vi "Append Waveform Properties to TDMS Channels.vi"(8 "error in":errorcluster, 10 "File Log Spec In":T1 {"File Node Ref" format="%.0x"}, 11 "TDMS File In":refnum<k34>) -> (0 "error out":errorcluster, 2 "File Log Spec":T1 {"File Node Ref" format="%.0x"}, 3 "TDMS File Out":refnum<k34>)   [LabVIEW 2027, in "Embedded Data Logger Engine.lvlib"]
uses:
  Embedded Data Logger Engine.lvlib
  File Logging Specification.ctl
  Group Logging Specification.ctl
  Group Buffer Data.ctl
  Property Specification.ctl
  <vilib>/NI VeriStand/Custom Device API/Custom Device Item Ref.ctl
  Shared/Segment Files By.ctl
  Logging State.ctl
  <vilib>/NI VeriStand/Custom Device API/Custom Device API.lvlib
  Shared/Embedded Data Logger Shared.lvlib
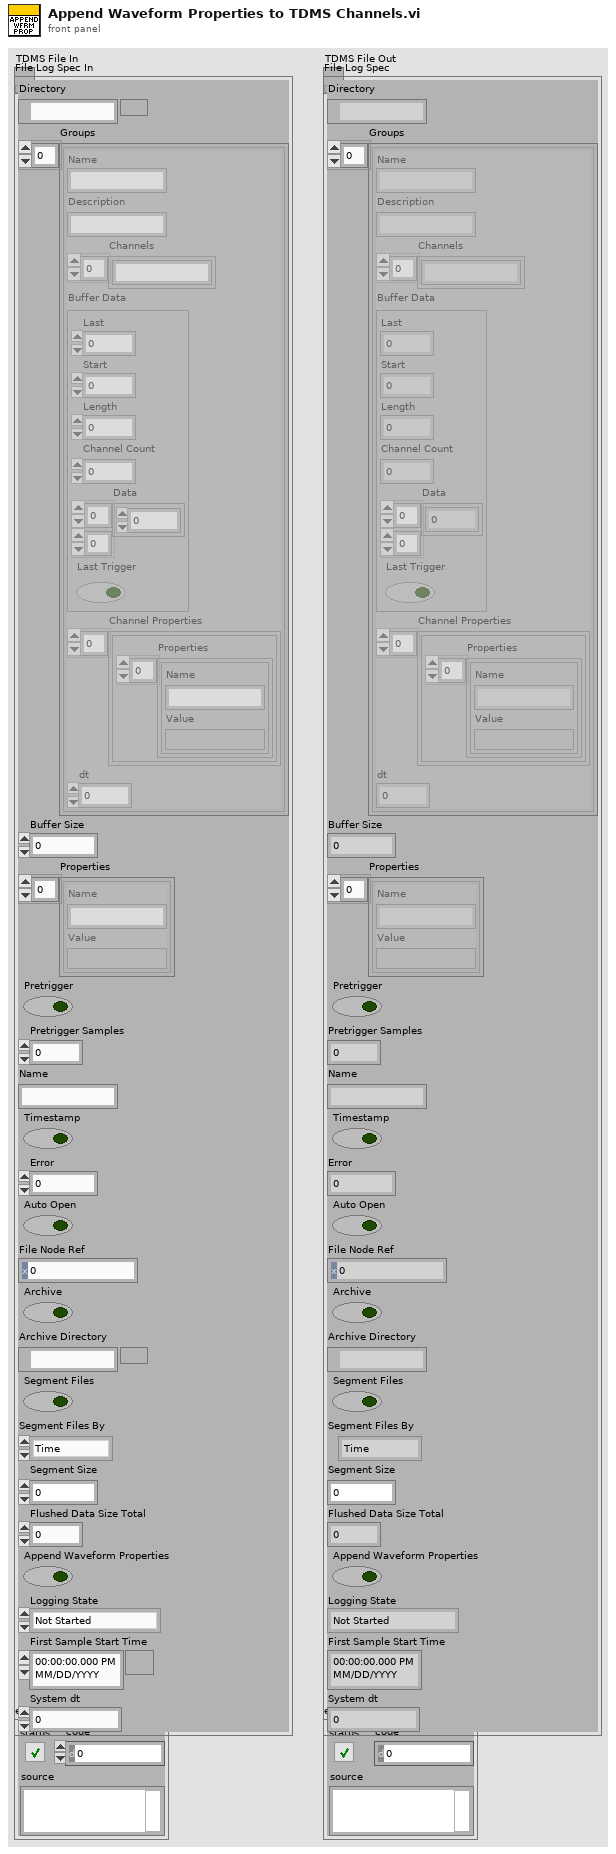
[diagram p1: front panel]
types:
  T1 = typedef "Embedded Data Logger Engine.lvlib/File Logging Specification.ctl" = cluster{"Directory":path, "Groups":T2[], "Buffer Size":i32, "Properties":T4[], "Pretrigger":bool, "Pretrigger Samples":i32, "Name":string, "Timestamp":bool, "Error":i32, "Auto Open":bool, "File Node Ref":T5, "Archive":bool, "Archive Directory":path, "Segment Files":bool, "Segment Files By":T6, "Segment Size":u32, "Flushed Data Size Total":u32, "Append Waveform Properties":bool, "Logging State":T7, "First Sample Start Time":timestamp, "System dt":dbl}
  T2 = typedef "Embedded Data Logger Engine.lvlib/Group Logging Specification.ctl" = cluster{"Name":string, "Description":string, "Channels":string[], "Buffer Data":T3, "Channel Properties":cluster{"Properties":T4[]}[], "dt":dbl}
  T3 = typedef "Embedded Data Logger Engine.lvlib/Group Buffer Data.ctl" = cluster{"Last":i32, "Start":i32, "Length":i32, "Channel Count":i32, "Data":dbl[][], "Last Trigger":bool}
  T4 = typedef "Embedded Data Logger Engine.lvlib/Property Specification.ctl" = cluster{"Name":string, "Value":variant}
  T5 = typedef "Custom Device API.lvlib/Custom Device Item Ref.ctl" = u64
  T6 = typedef "Embedded Data Logger Shared.lvlib/Segment Files By.ctl" = enum16{"Time", "Size"}
  T7 = typedef "Embedded Data Logger Engine.lvlib/Logging State.ctl" = enum16{"Not Started", "Continous Logging", "Paused", "Discontinous Logging"}
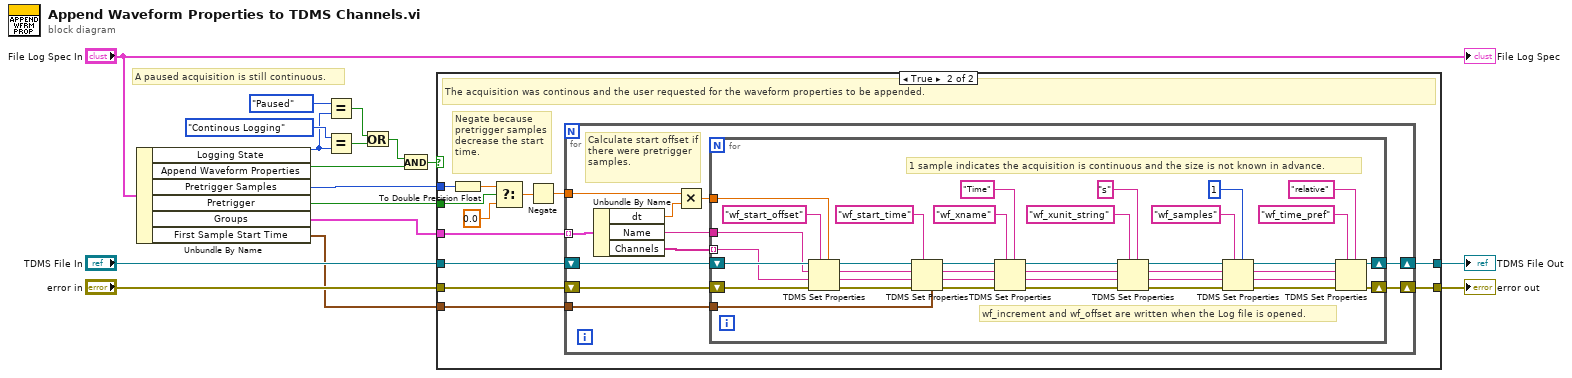
[diagram p0: block diagram]
diagram:
  # "A paused acquisition is still continuous."
  n1 = Unbundle By Name("File Log Spec In") -> ("Logging State"=w2:T7, "Append Waveform Properties"=w11:bool, "Pretrigger Samples"=w7:i32, "Pretrigger"=w8:bool, "Groups"=w9:T2[], "First Sample Start Time"=w6:timestamp)
  n2 = Equal?(x=Logging_State."Paused", y=w2) -> (x = y?=w3:bool)
  n3 = Equal?(x=Logging_State."Continous Logging" ("y"), y=w2) -> (x = y?=w4:bool)
  n4 = Or(x=w3, y=w4) -> (x .or. y?=w5:bool)
  n5 = And(x=w5, y=w11) -> (x .and. y?=w12:bool)
  n6 = case shown="True" w12 {
    tunnel: "error in" -> [w18 w31]
    tunnel: "TDMS File In" -> [w19 w30]
    tunnel: [w18 w29] -> w15
    tunnel: [w19 w28] -> w14
    tunnel: w9 -> [_ w27]
    tunnel: w8 -> [_ w26]
    tunnel: w7 -> [_ w25]
    tunnel: w6 -> [_ w20]
    frame False {
      # "The acquisition was discontinuous or the waveform properties were not requested."
    }
    frame True {
      # "Negate because pretrigger samples decrease the start time."
      # "The acquisition was continous and the user requested for the waveform properties to be appended."
      n7 = To Double Precision Float(number=w25) -> (double precision float=w24:dbl)
      n8 = Select(t=w24, s=w26, f=0.0) -> (s? t:f=w22:dbl)
      n9 = Negate(x=w22) -> (-x=w21:dbl)
      n10 = for {
        shift-right: [w42] -> w29
        shift-left: w31 -> [w38]
        shift-right: [w41] -> w28
        shift-left: w30 -> [w39]
        tunnel: w27 -> [w40] mode=indexing
        tunnel: w21 -> [w35]
        tunnel: w20 -> [w34]
        # "Calculate start offset if there were pretrigger samples."
        n11 = Unbundle By Name(w40) -> ("dt"=w32:dbl, "Name"=w33:string, "Channels"=w37:string[])
        n12 = Multiply(x=w35, y=w32) -> (x*y=w36:dbl)
        n13 = for {
          shift-right: [w57] -> w42
          shift-left: w38 -> [w59]
          shift-right: [w56] -> w41
          shift-left: w39 -> [w58]
          tunnel: w37 -> [w55] mode=indexing
          tunnel: w36 -> [w54]
          tunnel: w34 -> [w44]
          tunnel: w33 -> [w43]
          # "wf_increment and wf_offset are written when the Log file is opened."
          # "1 sample indicates the acquisition is continuous and the size is not known in advance."
          n14 = TDMS Set Properties(5:w54, 7:"wf_start_offset" ("group name in (Untitled)"), 8:w59, 9:w55, 10:w43, 11:w58) -> (0:w51:errorcluster, 1:w47:string, 2:w48:string, 3:w52:refnum<k34>)
          n15 = TDMS Set Properties(5:w44, 7:"wf_start_time" ("group name in (Untitled)"), 8:w51, 9:w47, 10:w48, 11:w52) -> (0:w49:errorcluster, 1:w45:string, 2:w46:string, 3:w50:refnum<k34>)
          n16 = TDMS Set Properties(5:"Time" ("group name in (Untitled)"), 7:"wf_xname" ("group name in (Untitled)"), 8:w49, 9:w45, 10:w46, 11:w50) -> (0:w76:errorcluster, 1:w72:string, 2:w73:string, 3:w77:refnum<k34>)
          n17 = TDMS Set Properties(5:"s" ("group name in (Untitled)"), 7:"wf_xunit_string" ("group name in (Untitled)"), 8:w76, 9:w72, 10:w73, 11:w77) -> (0:w70:errorcluster, 1:w64:string, 2:w65:string, 3:w71:refnum<k34>)
          n18 = TDMS Set Properties(5:1, 7:"wf_samples" ("group name in (Untitled)"), 8:w70, 9:w64, 10:w65, 11:w71) -> (0:w68:errorcluster, 1:w62:string, 2:w63:string, 3:w69:refnum<k34>)
          n19 = TDMS Set Properties(5:"relative" ("group name in (Untitled)"), 7:"wf_time_pref" ("group name in (Untitled)"), 8:w68, 9:w62, 10:w63, 11:w69) -> (0:w57:errorcluster, 3:w56:refnum<k34>)  [unwired: 2 out]
        }
      }
    }
  }
  "error out" <- w15
  "TDMS File Out" <- w14
  "File Log Spec" <- "File Log Spec In"
